vi "Display Date and Time.vi"() -> (0 "Time":string, 3 "Date":string)   [LabVIEW 2023, in "GUI.lvlib"]
uses:
  GUI.lvlib
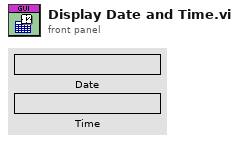
[diagram p1: front panel]
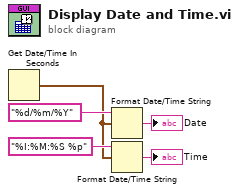
[diagram p0: block diagram]
diagram:
  n1 = Get Date/Time In Seconds() -> (seconds since 1Jan1904=w3:timestamp)
  n2 = Format Date/Time String(time format string (%c)="%d/%m/%Y", seconds (now)=w3) -> (date/time string=→"Date":string)  [unwired: 1 in]
  n3 = Format Date/Time String(time format string (%c)="%I:%M:%S %p", seconds (now)=w3) -> (date/time string=→"Time":string)  [unwired: 1 in]
